vi "Trial Fraction.vi"(7 "Trial In Progress IN":T1, 10 "cur_trial_dist":dbl format="%.1f", 11 "Time into Trial":dbl) -> (1 "Trial Fraction":dbl, 2 "Timeout Timer":dbl, 3 "Timeout?":bool)   [LabVIEW 2018]
uses:
  controls/Trial Config Settings.ctl
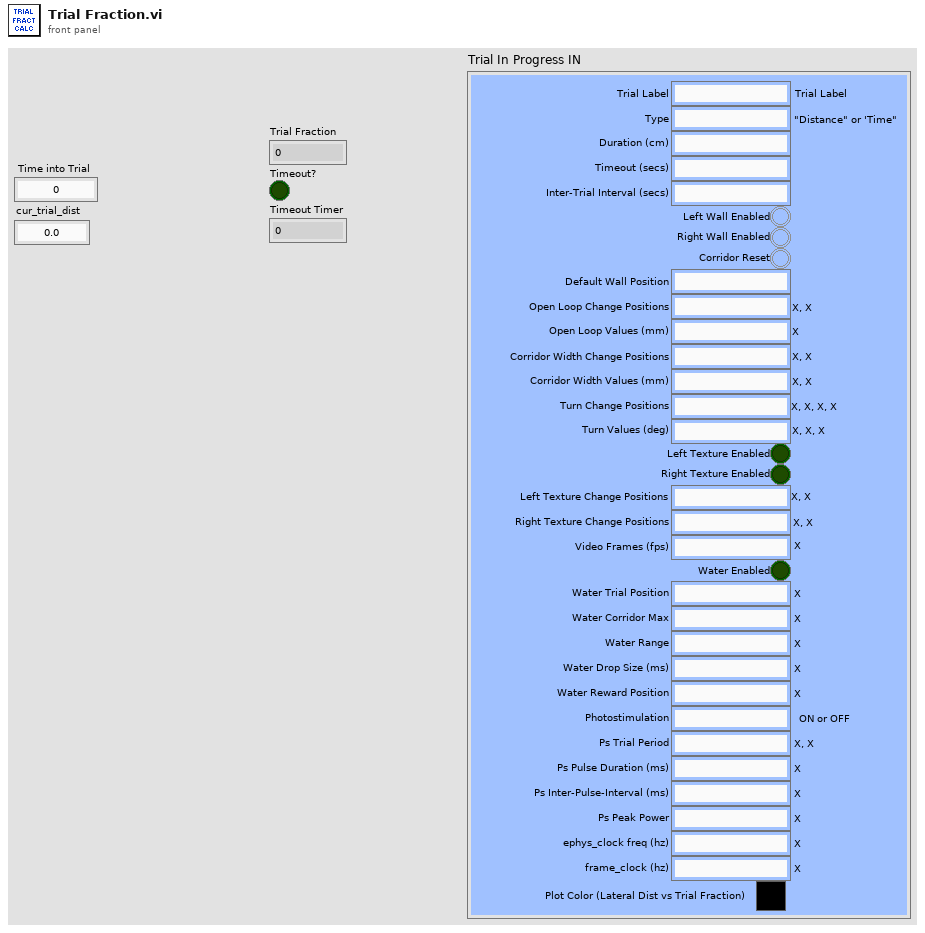
[diagram p1: front panel]
types:
  T1 = typedef "Trial Config Settings.ctl" = cluster{"Trial Label":string, "Type":string, "Timeout (secs)":string, "Inter-Trial Interval (secs)":string, "Left Wall Enabled":bool, "Right Wall Enabled":bool, "Corridor Reset":bool, "Default Wall Position":string, "Open Loop Change Positions":string, "Open Loop Values (mm)":string, "Corridor Width Change Positions":string, "Corridor Width Values (mm) ":string, "Turn Change Positions":string, "Turn Values (deg)":string, "Left Texture Change Positions":string, "Right Texture Change Positions":string, "Video Frames (fps)":string, "Water Enabled":bool, "Water Trial Position":string, "Photostimulation":string, "Water Corridor Max":string, "Water Range":string, "Water Drop Size (ms)":string, "Water Reward Position":string, "Duration (cm)":string, "Left Texture Enabled":bool, "Right Texture Enabled":bool, "Ps Trial Period":string, "Ps Inter-Pulse-Interval (ms)":string, "Ps Peak Power":string, "Ps Pulse Duration (ms)":string, "ephys_clock freq (hz)":string, "frame_clock (hz)":string, "Plot Color (Lateral Dist vs Trial Fraction)":u32}
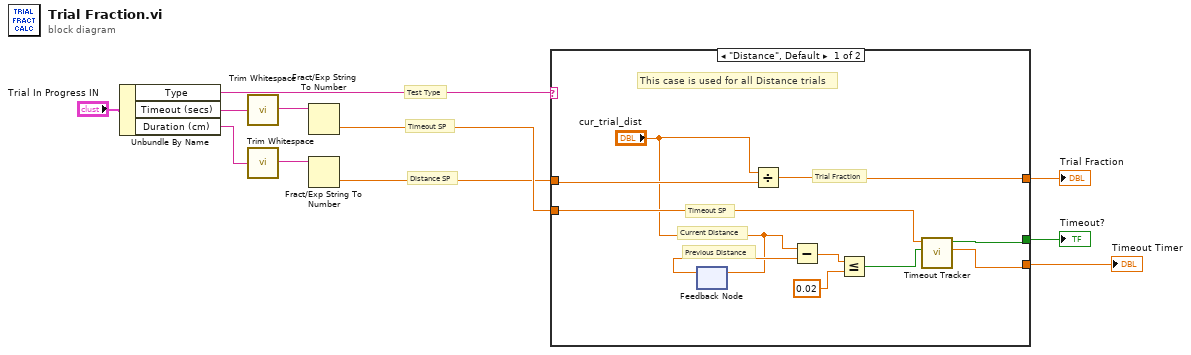
[diagram p0: block diagram]
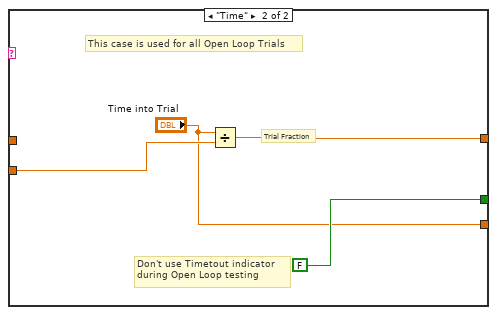
[diagram p2: hidden frame]
diagram:
  # "Test Type"
  # "Timeout SP"
  # "Distance SP"
  n1 = Unbundle By Name("Trial In Progress IN") -> ("Type"=w7:string, "Timeout (secs)"=w6:string, "Duration (cm)"=w2:string)
  n2 = call <vilib>:"Trim Whitespace.vi"("string"=w6) -> ("trimmed string"=w5:string)  [unwired: 1 in]
  n3 = call <vilib>:"Trim Whitespace.vi"("string"=w2) -> ("trimmed string"=w3:string)  [unwired: 1 in]
  n4 = Fract/Exp String To Number(string=w5) -> (number=w4:dbl)  [unwired: 3 in, 1 out]
  n5 = Fract/Exp String To Number(string=w3) -> (number=w1:dbl)  [unwired: 3 in, 1 out]
  n6 = case shown="\"Distance\", Default" w7 {
    tunnel: [w21 w25] -> w11
    tunnel: w4 -> [w20 w24]
    tunnel: [w19 FALSE ("Timeout")] -> w10
    tunnel: [w18 "Time into Trial"] -> w9
    tunnel: w1 -> [w17 _]
    frame "Distance", Default {
      # "Trial Fraction"
      # "This case is used for all Distance trials"
      # "Timeout SP"
      # "Current Distance"
      # "Previous Distance"
      n7 = feedback #1() -> (w16:dbl)  [unwired: 1 in]
      n8 = feedback-in #1("cur_trial_dist") -> ()
      n9 = Divide(x="cur_trial_dist", y=w17) -> (x/y=w21:dbl)
      n10 = Subtract(x="cur_trial_dist", y=w16) -> (x-y=w13:dbl)
      n11 = Less Or Equal?(x=w13, y=0.02) -> (x <= y?=w14:bool)
      n12 = call "Timeout Tracker.vi"("Mouse Not Moving?"=w14, "Timeout SP"=w20) -> ("Timeout Timer"=w18:dbl, "Timeout"=w19:bool)  [unwired: 8 in]
    }
    frame "Time" {
      # "Trial Fraction"
      # "This case is used for all Open Loop Trials"
      # "Don't use Timetout indicator\nduring Open Loop testing"
      n13 = Divide(x="Time into Trial", y=w24) -> (x/y=w25:dbl)
    }
  }
  "Trial Fraction" <- w11
  "Timeout?" <- w10
  "Timeout Timer" <- w9
